vi "setup.vi"(7 "LabVIEW Web Service Request":refnum<class "Web Request.lvclass">, 10 "back_url":string, 11 "context_id":string) -> (3 "url":string)   [LabVIEW 2013]
uses:
  <vilib>/wsapi/Web Request.lvclass
  <vilib>/Utility/config.llb/Read Key (U32).vi
  <vilib>/Utility/config.llb/Write Key (U32).vi
  <vilib>/Utility/config.llb/Write Key (String).vi
  <vilib>/Utility/config.llb/NI_LVConfig.lvlib
panel:
  out "date":string
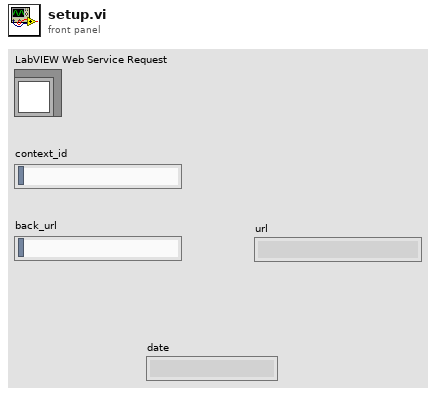
[diagram p1: front panel]
types:
  T1 = typedef "NI_LVConfig.lvlib/Config Data RefNum.ctl" = refnum<k1>
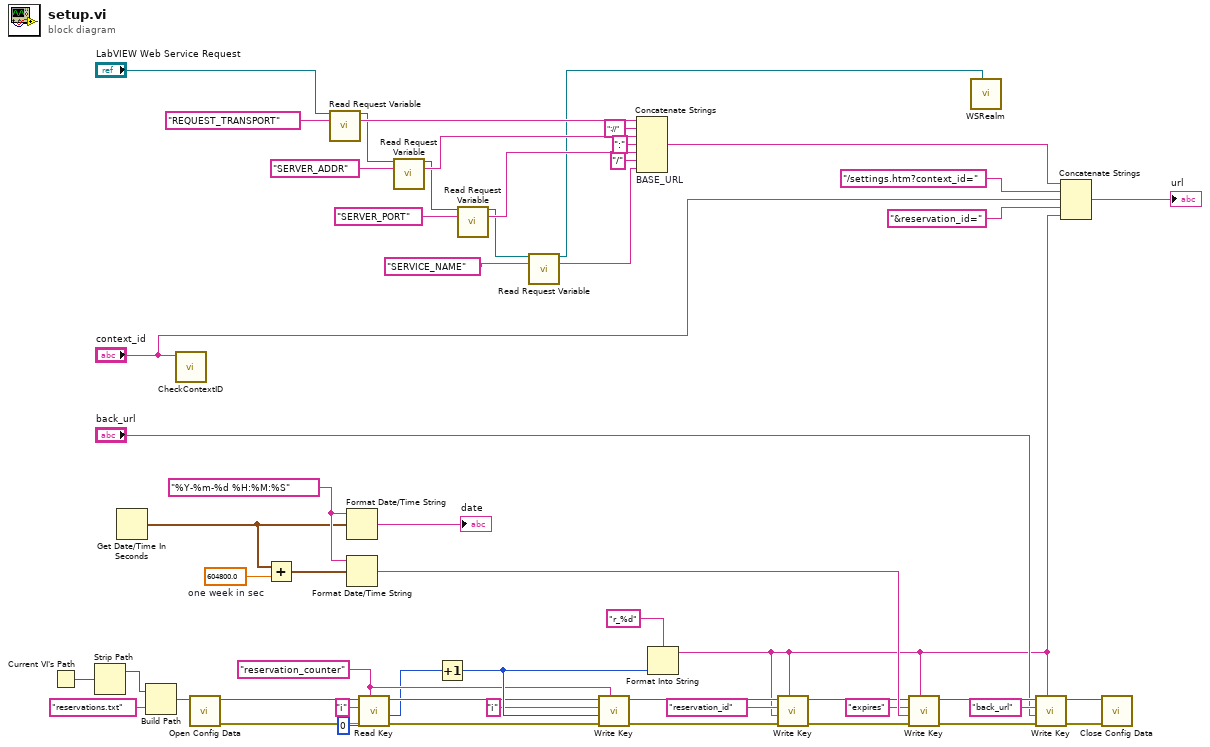
[diagram p0: block diagram]
diagram:
  w40 = "reservation_counter" ("section")
  w24 = 604800.0  # one week in sec
  w26 = "%Y-%m-%d %H:%M:%S" ("time format string (%c)")
  n1 = Current VI's Path() -> (path=w11:path)
  n2 = Strip Path(path=w11) -> (stripped path=w12:path)  [unwired: 1 out]
  n3 = Get Date/Time In Seconds() -> (seconds since 1Jan1904=w23:timestamp)
  n4 = Build Path(base path=w12, name or relative path="reservations.txt") -> (appended path=w14:path)
  n5 = call "CheckContextID.vi"("context_id"="context_id") -> ()  [unwired: 10 in, 1 out]
  n6 = call <vilib>:"Open Config Data.vi"("configuration file path"=w14) -> ("error out"=w30:errorcluster, "refnum"=w29:T1)  [unwired: 8 in, 1 out]
  n7 = Add(x=w23, y=w24) -> (x+y=w27:timestamp)
  n8 = call <vilib>:"Read Request Variable.vi"("LabVIEW Web Service Request"="LabVIEW Web Service Request", "variable name"="REQUEST_TRANSPORT") -> ("LabVIEW Web Service Request out"=w47:refnum<class "Web Request.lvclass">, "value"=w49:string)  [unwired: 11 in, 1 out]
  n9 = Format Date/Time String(time format string (%c)=w26, seconds (now)=w23) -> (date/time string=→"date":string)  [unwired: 1 in]
  n10 = Format Date/Time String(time format string (%c)=w26, seconds (now)=w27) -> (date/time string=w28:string)  [unwired: 1 in]
  n11 = call-poly <vilib>:"Read Key.vi"("section"=w40, "error in (no error)"=w30, "default value"=u32 0, "key"="i", "refnum"=w29) -> ("error out"=w37:errorcluster, "value"=w33:u32, "refnum out"=w38:T1)  [unwired: 3 in, 1 out]
  n12 = call <vilib>:"Read Request Variable.vi"("LabVIEW Web Service Request"=w47, "variable name"="SERVER_ADDR") -> ("LabVIEW Web Service Request out"=w48:refnum<class "Web Request.lvclass">, "value"=w51:string)  [unwired: 11 in, 1 out]
  n13 = Increment(x=w33) -> (x+1=w41:u32)
  n14 = call <vilib>:"Read Request Variable.vi"("LabVIEW Web Service Request"=w48, "variable name"="SERVER_PORT") -> ("LabVIEW Web Service Request out"=w4:refnum<class "Web Request.lvclass">, "value"=w53:string)  [unwired: 11 in, 1 out]
  n15 = call <vilib>:"Read Request Variable.vi"("LabVIEW Web Service Request"=w4, "variable name"="SERVICE_NAME") -> ("LabVIEW Web Service Request out"=w3:refnum<class "Web Request.lvclass">, "value"=w2:string)  [unwired: 11 in, 1 out]
  n16 = call-poly <vilib>:"Write Key.vi"("section"=w40, "error in (no error)"=w37, "value"=w41, "key"="i", "refnum"=w38) -> ("error out"=w36:errorcluster, "refnum out"=w35:T1)  [unwired: 4 in, 1 out]
  n17 = Concatenate Strings "BASE_URL"(w49, "://" ("string"), w51, ":" ("string"), w53, "/" ("string"), w2) -> (w54:string)
  n18 = Format Into String(format string="r_%d", w41) -> (resulting string=w1:string)  [unwired: 2 in, 1 out]
  n19 = call-poly <vilib>:"Write Key.vi"("section"=w1, "error in (no error)"=w36, "value"=w1, "key"="reservation_id", "refnum"=w35) -> ("error out"=w16:errorcluster, "refnum out"=w15:T1)  [unwired: 4 in, 1 out]
  n20 = call-poly <vilib>:"Write Key.vi"("section"=w1, "error in (no error)"=w16, "value"=w28, "key"="expires", "refnum"=w15) -> ("error out"=w18:errorcluster, "refnum out"=w17:T1)  [unwired: 4 in, 1 out]
  n21 = call "WSRealm.vi"("LabVIEW Web Service Request"=w3) -> ()  [unwired: 11 in]
  n22 = call-poly <vilib>:"Write Key.vi"("section"=w1, "error in (no error)"=w18, "value"="back_url", "key"="back_url", "refnum"=w17) -> ("error out"=w20:errorcluster, "refnum out"=w19:T1)  [unwired: 4 in, 1 out]
  n23 = Concatenate Strings(w54, "/settings.htm?context_id=" ("string"), "context_id", "&reservation_id=" ("string"), w1) -> (→"url":string)
  n24 = call <vilib>:"Close Config Data.vi"("error in (no error)"=w20, "refnum"=w19) -> ()  [unwired: 8 in, 2 out]
